vi "Read Cell font.vi"(8 "error in (no error)":errorcluster, 11 "DatagridElement in":refnum<class "DatagridElement.lvclass">) -> (0 "error out":errorcluster, 2 "Font":T1, 3 "DatagridElement out":refnum<class "DatagridElement.lvclass">)   [LabVIEW 2020, in "D Datagrid Library.lvlib" / "DatagridElement.lvclass"]
uses:
  DatagridElement.lvclass
  DatagridElement.lvclass/DatagridElement.ctl
  <vilib>/Utility/miscctls.llb/LVFontTypeDef.ctl
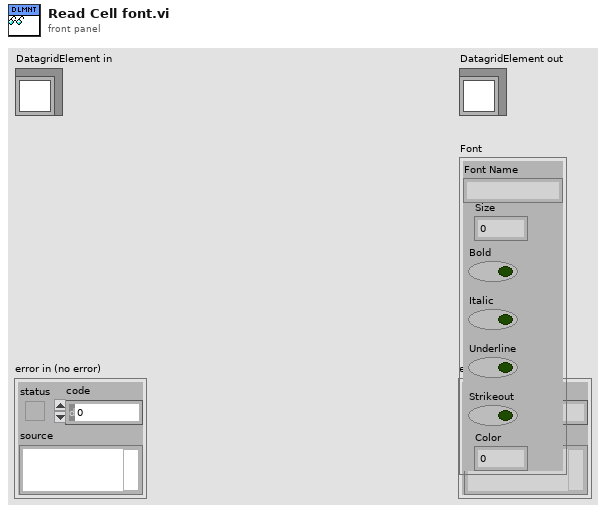
[diagram p1: front panel]
types:
  T1 = typedef "LVFontTypeDef.ctl" = cluster{"Font Name":string, "Size":u16, "Bold":bool, "Italic":bool, "Underline":bool, "Strikeout":bool, "Color":u32}
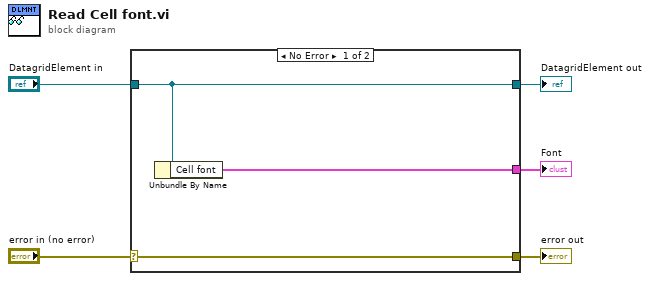
[diagram p0: block diagram]
diagram:
  n1 = case shown="No Error" "error in (no error)" {
    selector: "error in (no error)" -> [w8 w9]
    tunnel: [w8 w9] -> w4
    tunnel: [w7 w10] -> w2
    tunnel: "DatagridElement in" -> [w7 w10]
    tunnel: [w6 _] -> w1
    frame No Error {
      n2 = Unbundle By Name(w7) -> ("Cell font"=w6:T1)
    }
    frame Error {
    }
  }
  "error out" <- w4
  "DatagridElement out" <- w2
  "Font" <- w1
